vi "周围状态个数.vi"(2 "索引":i32, 3 "地图":i32[][](array[numeric])) -> (0 "未标记数":i32, 1 "标记数":i32)   [LabVIEW 2017]
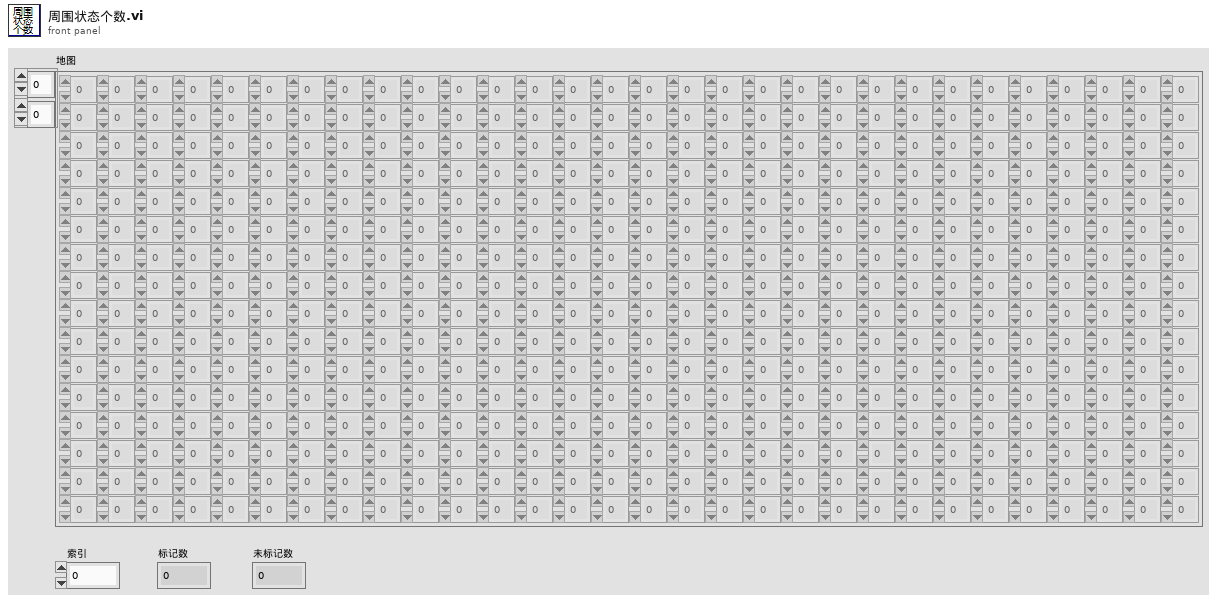
[diagram p1: front panel]
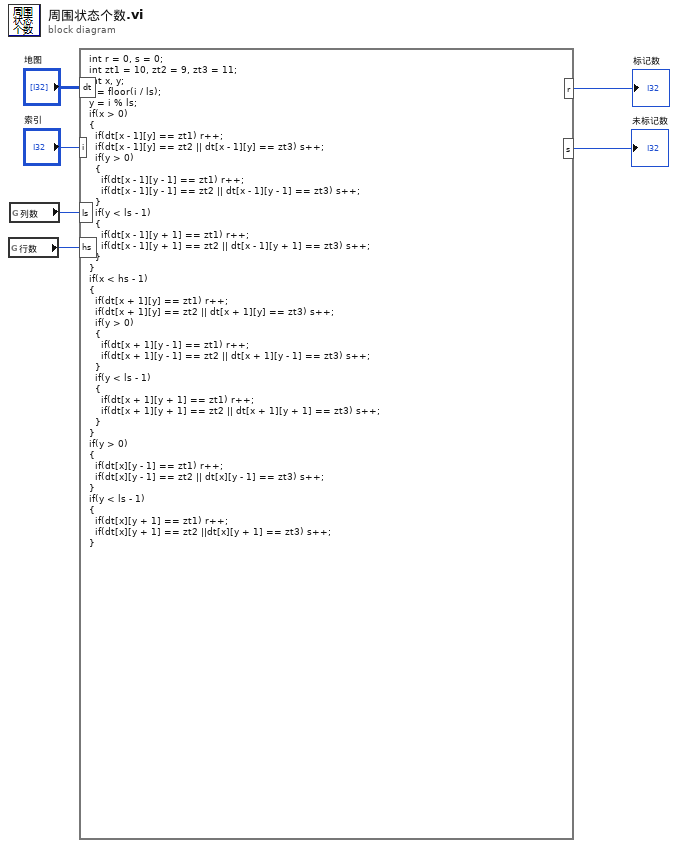
[diagram p0: block diagram]
diagram:
  n1 = global read "全局变量.vi" "行数"() -> (w1:i32)
  n2 = global read "全局变量.vi" "列数"() -> (w2:i32)
  n3 = formula code="int r = 0, s = 0;\nint zt1 = 10, zt2 = 9, zt3 = 11;\nint x, y;\nx = floor(i / ls);\ny = i % ls;\nif(x > 0)\n{\n  if(dt[x - 1][y] == zt1) r++;\n  if(dt[x - 1][y] == zt2 || dt[x - 1][y] == zt3) s++;\n  if(y > 0)\n  {\n    if(dt[x - 1][y - 1] == zt1) r++;\n    if(dt[x - 1][y - 1] == zt2 || dt[x - 1][y - 1] == zt3) s++;\n  }\n  if(y < ls - 1)\n  {\n    if(dt[x - 1][y + 1] == zt1) r++;\n    if(dt[x - 1][y + 1] == zt2 || dt[x - 1][y + 1] == zt3) s++;\n  }\n}\nif(x < hs - 1)\n{\n  if(dt[x + 1][y] == zt1) r++;\n  if(dt[x + 1][y] == zt2 || dt[x + 1][y] == zt3) s++;\n  if(y > 0)\n  {\n    if(dt[x + 1][y - 1] == zt1) r++;\n    if(dt[x + 1][y - 1] == zt2 || dt[x + 1][y - 1] == zt3) s++;\n  }\n  if(y < ls - 1)\n  {\n    if(dt[x + 1][y + 1] == zt1) r++;\n    if(dt[x + 1][y + 1] == zt2 || dt[x + 1][y + 1] == zt3) s++;\n  }\n}\nif(y > 0)\n{\n  if(dt[x][y - 1] == zt1) r++;\n  if(dt[x][y - 1] == zt2 || dt[x][y - 1] == zt3) s++;\n}\nif(y < ls - 1)\n{\n  if(dt[x][y + 1] == zt1) r++;\n  if(dt[x][y + 1] == zt2 ||dt[x][y + 1] == zt3) s++;\n}"("dt"="地图", "i"="索引", "ls"=w2, "hs"=w1) -> ("s"=→"未标记数":i32, "r"=→"标记数":i32)
